vi "Vision Processing.vi"(4 "error in (no error)":errorcluster) -> ()   [LabVIEW 2012]
doc: "This VI runs in parallel to other tasks. It gets images from the camera, processes them for color or shape and use that information to affect robot behavior."
uses:
  Robot Global Data.vi
  <vilib>/vision/NI_Vision_Development_Module.lvlib
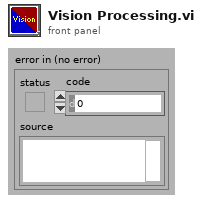
[diagram p1: front panel]
types:
  T1 = typedef "Image Type" = u32
  T2 = typedef "WPI_CameraDevRef.ctl" = cluster{"Camera Address":string, "CameraStatus":errorcluster, "Acquire Image Notifier":refnum<notifier>}
  T3 = typedef "IMAQ Image.ctl" = refnum<image>
  T4 = cluster{"Rect Coverage":dbl, "X Edge Strength":dbl, "Y Edge Strength":dbl, "Center":dbl, "Outer":dbl}
  T5 = cluster{"Position":cluster{"X":dbl, "Y":dbl}, "Distance (ft)":dbl, "Center":bool}[]
  T6 = typedef "WPI_CameraImageSize.ctl" = enum16{"640x480", "320x240", "160x120"}
  T7 = cluster{cluster{"Left":dbl, "Top":dbl, "Right":dbl, "Bottom":dbl}, "Scores":dbl[], cluster{"Long":dbl, "Short":dbl}}[]
  T8 = cluster{"Target Center (-1 to 1)":cluster{"X":dbl, "Y":dbl}, "Distance (ft)":dbl, "Center Target":bool}
  T9 = cluster{"Target Center (-1 to 1)":cluster{"X":dbl, "Y":dbl}, "Distance (ft)":dbl, "Center Target":bool}[]
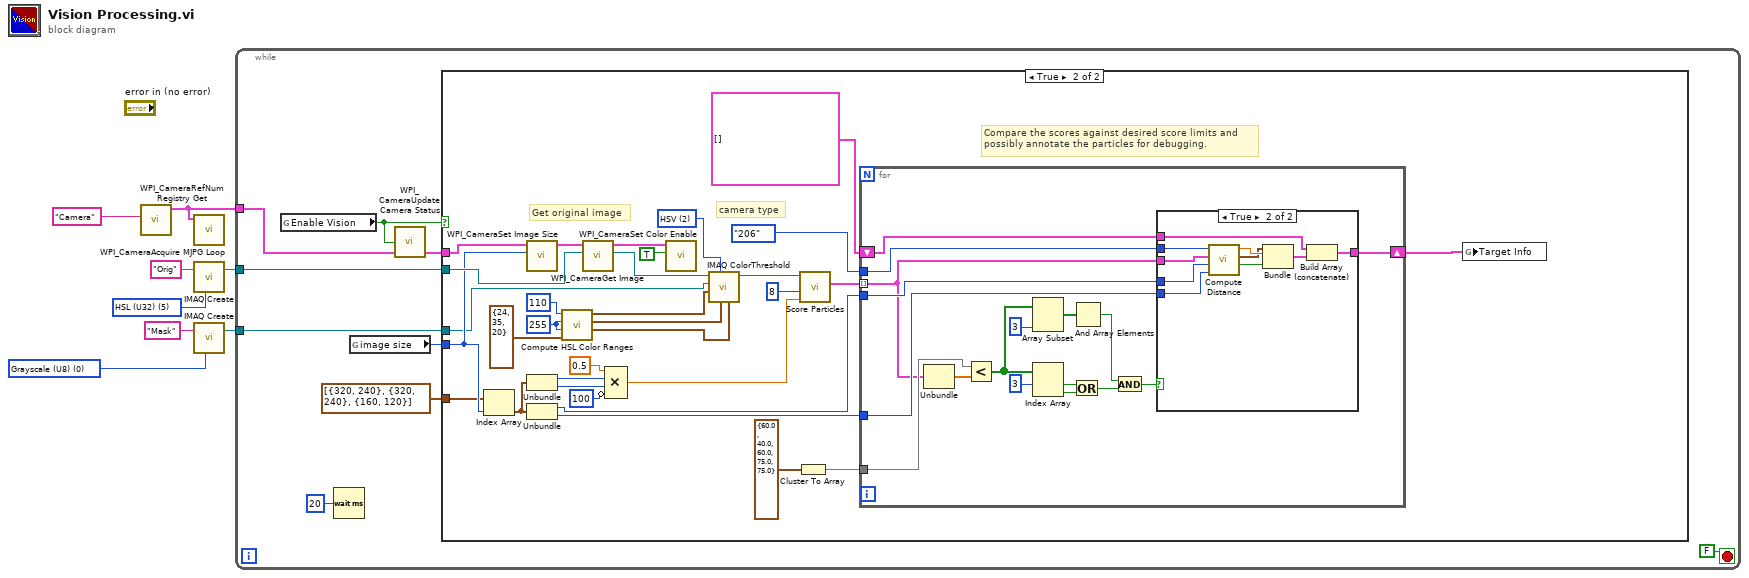
[diagram p0: block diagram]
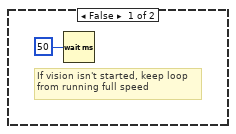
[diagram p2: hidden frame]
diagram:
  w4 = T1 0 items=["Grayscale (U8)", "Grayscale (I16)", "Grayscale (SGL)", "Complex (CSG)", "RGB (U32)", "HSL (U32)", "RGB (U64)", "Grayscale (U16)"] ("Image Type")
  w7 = T1 5 items=["Grayscale (U8)", "Grayscale (I16)", "Grayscale (SGL)", "Complex (CSG)", "RGB (U32)", "HSL (U32)", "RGB (U64)", "Grayscale (U16)"] ("Image Type")
  n1 = call <vilib>:"WPI_CameraRefNum Registry Get.vi"("refnum name"="Camera") -> ("CameraDevRef"=w5:T2)  [unwired: 9 in, 1 out]
  n2 = call <vilib>:"WPI_CameraAcquire MJPG Loop.vi"("CameraDevRef"=w5) -> ()  [unwired: 11 in]
  n3 = call "IMAQ Create"("Image Name"="Orig", "Image Type"=w7) -> ("New Image"=w6:T3)  [unwired: 2 in, 2 out]
  n4 = call "IMAQ Create"("Image Name"="Mask", "Image Type"=w4) -> ("New Image"=w2:T3)  [unwired: 2 in, 2 out]
  n5 = while {
    tunnel: w6 -> [w16]
    tunnel: w5 -> [w15]
    tunnel: w2 -> [w11]
    stop <- FALSE stop-if-true
    n6 = global read "Robot Global Data.vi" "Enable Vision"() -> (w13:bool)
    n7 = Wait (ms)(milliseconds to wait=u32 20) -> ()  [unwired: 1 out]
    n8 = global read "Robot Global Data.vi" "image size"() -> (w12:T6)
    n9 = call <vilib>:"WPI_CameraUpdate Camera Status.vi"("CameraDevRef In"=w15, "Enable Vision"=w13) -> ("CameraDevRef Out"=w14:T2)  [unwired: 3 in]
    n10 = case shown="True" w13 {
      tunnel: w16 -> [_ w47]
      tunnel: w14 -> [_ w44]
      tunnel: w12 -> [_ w42]
      tunnel: w11 -> [_ w38]
      tunnel: cluster{i32, i32}[] [{320, 240}, {320, 240}, {160, 120}] -> [_ w41]
      frame False {
        # "If vision isn't started, keep loop\nfrom running full speed"
        n11 = Wait (ms)(milliseconds to wait=u32 50) -> ()  [unwired: 1 out]
      }
      frame True {
        w22 = 255
        w28 = u16 2 items=["RGB", "HSL", "HSV", "HSI"] ("Color Mode")
        # "camera type"
        # "Compare the scores against desired score limits and\npossibly annotate the particles for debugging."
        # "Get original image"
        n12 = Index Array(array=w41, index=w42) -> (element=w19:cluster{i32, i32})
        n13 = call <vilib>:"WPI_CameraSet Image Size.vi"("Image Size"=w42, "CameraDevRef"=w44) -> ("CameraDevRef Out"=w45:T2)  [unwired: 8 in, 1 out]
        n14 = Unbundle(w19) -> (w34:i32, w33:i32)
        n15 = Unbundle(w19) -> (w40:i32, w39:i32)
        n16 = call "Compute HSL Color Ranges.vi"("Margins"=cluster{"Hue":i32, "Sat":i32, "Val":i32} {"Hue"=24, "Sat"=35, "Val"=20}, "Luminance"=w22, "Saturation"=w22, "Hue"=110) -> ("Lum Range"=w25:cluster{i32, i32}, "Sat Range"=w27:cluster{i32, i32}, "Hue Range"=w24:cluster{i32, i32})  [unwired: 5 in]
        n17 = call <vilib>:"WPI_CameraGet Image.vi"("Image"=w47, "CameraDevRef"=w45) -> ("Image Out"=w37:T3, "CameraDevRef Out"=w46:T2)  [unwired: 7 in, 1 out]
        n18 = Compound Arithmetic op=MULTIPLY(0.5, w34, w33, invert 100 ("length")) -> (w31:dbl)
        n19 = call <vilib>:"WPI_CameraSet Color Enable.vi"("Color Enabled"=TRUE, "CameraDevRef"=w46) -> ()  [unwired: 8 in, 2 out]
        n20 = call "IMAQ ColorThreshold"("Blue or Luma or Val or Inten Range"=w25, "Green or Sat Range"=w27, "Color Mode"=w28, "Red or Hue Range"=w24, "Image Dst"=w38, "Image Src"=w37) -> ("Image Dst Out"=w43:T3)  [unwired: 4 in, 1 out]
        n21 = Cluster To Array(cluster=T4 {"Rect Coverage"=60.0, "X Edge Strength"=40.0, "Y Edge Strength"=60.0, "Center"=75.0, "Outer"=75.0} ("Score Limits")) -> (array=w48:dbl[])
        n22 = call "Score Particles.vi"("Area Size Limit"=w31, "Particle Count Limit"=8, "Image Refnum in"=w43) -> ("Scored Particle Info"=w49:T7)  [unwired: 7 in, 1 out]
        n23 = for {
          shift-right: [w66] -> w35
          shift-left: T5 [] -> [w67]
          tunnel: w40 -> [w65]
          tunnel: w49 -> [w60] mode=indexing
          tunnel: w48 -> [w62]
          tunnel: enum16{"206", "1011"}."206" -> [w64]
          tunnel: w39 -> [w61]
          n24 = Unbundle(w60) -> ("Scores"=w63:dbl[])  [unwired: 2 out]
          n25 = Less?(x=w62, y=w63) -> (x < y?=w52:bool[])
          n26 = Array Subset(array=w52, length=3) -> (w54:bool[])  [unwired: 1 in]
          n27 = Index Array(array=w52, index #1=3 ("length")) -> (element #1=w56:bool, element #2=w57:bool)  [unwired: 1 in]
          n28 = Or(x=w56, y=w57) -> (x .or. y?=w58:bool)
          n29 = And Array Elements(Boolean array=w54) -> (logical AND=w59:bool)
          n30 = And(x=w59, y=w58) -> (x .and. y?=w51:bool)
          n31 = case shown="True" w51 {
            tunnel: w67 -> [w68 w78]
            tunnel: [w68 w77] -> w66
            tunnel: w65 -> [_ w75]
            tunnel: w64 -> [_ w73]
            tunnel: w61 -> [_ w72]
            tunnel: w60 -> [_ w70]
            frame False {
            }
            frame True {
              n32 = call "Compute Distance.vi"("Y Image Resolution"=w72, "X Image Resolution"=w75, "Particle Scores"=w70, "Camera Type"=w73) -> ("Center Target"=w69:bool, "Target Center (-1 to 1)"=w71:cluster{"X":dbl, "Y":dbl}, "Distance (ft)"=w74:dbl)  [unwired: 5 in]
              n33 = Bundle("Target Center (-1 to 1)"=w71, "Distance (ft)"=w74, "Center Target"=w69) -> (w76:T8)  [unwired: 1 in]
              n34 = Build Array (concatenate)(w78, w76) -> (w77:T9)
            }
          }
        }
        n35 = global write "Robot Global Data.vi" "Target Info"(w35) -> ()
      }
    }
  }
